vi "App1_TempComp.vi"() -> ()   [LabVIEW 2022 SP3]
uses:
  <vilib>/DAQmx/read.llb/DAQmx Read (Analog DBL 1Chan 1Samp).vi
  <vilib>/DAQmx/miscellaneous.llb/DAQmx Fill In Error Info.vi
panel:
  out "27\n27":bool
  out "28":bool
  out "29":bool
  out "30":bool
  out "Waveform Chart":dbl(graph)
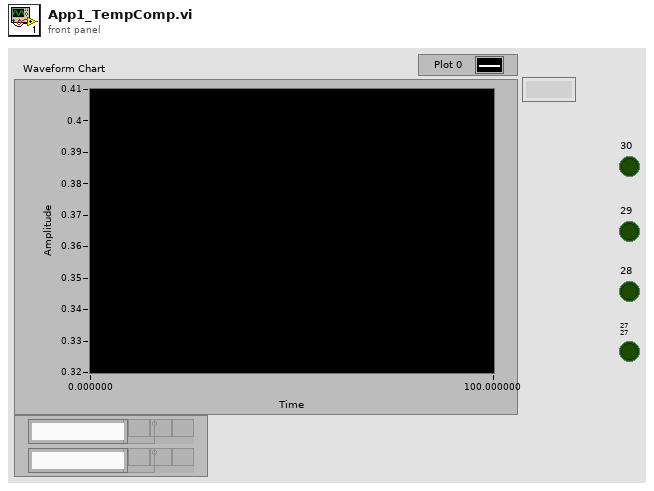
[diagram p1: front panel]
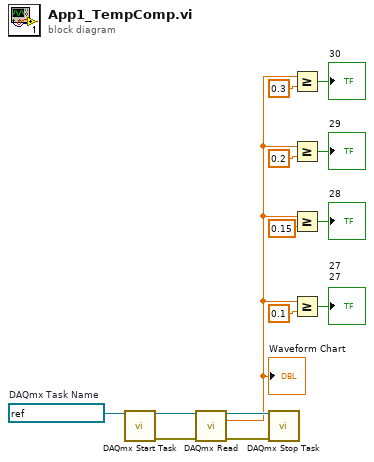
[diagram p0: block diagram]
diagram:
  w10 = refnum<k21> "Temp Sensor"  # DAQmx Task Name
  n1 = call <vilib>:"DAQmx Start Task.vi"("task/channels in"=w10) -> ("task out"=w12:refnum<k21>, "error out"=w14:errorcluster)  [unwired: 13 in]
  n2 = call-poly <vilib>:"DAQmx Read.vi"("task/channels in"=w12, "error in"=w14) -> ("task out"=w11:refnum<k21>, "data"=w1:dbl, "error out"=w13:errorcluster)  [unwired: 11 in]
  "Waveform Chart" <- w1
  n3 = call <vilib>:"DAQmx Stop Task.vi"("task/channels in"=w11, "error in"=w13) -> ()  [unwired: 12 in, 2 out]
  n4 = Greater Or Equal?(x=w1, y=0.3) -> (x >= y?=→"30":bool)
  n5 = Greater Or Equal?(x=w1, y=0.2) -> (x >= y?=→"29":bool)
  n6 = Greater Or Equal?(x=w1, y=0.15) -> (x >= y?=→"28":bool)
  n7 = Greater Or Equal?(x=w1, y=0.1) -> (x >= y?=→"27\n27":bool)
